vi "appendExptParam.vi"(8 "error in (no error)":errorcluster, 9 "value":variant, 10 "key":string, 11 "Inst.Transport in":refnum<class "Inst.Transport.lvclass">) -> (0 "error out":errorcluster, 3 "Inst.Transport out":refnum<class "Inst.Transport.lvclass">)   [LabVIEW 2019, in "Inst.Transport.lvclass"]
uses:
  Inst.Transport.lvclass
  Typedefs/Inst.Transport.PublicCommands--Enum.ctl
  e5f6a06c-75fd-45dd-8cd9-e6d3d0cfac2f.vi
  <vilib>/JDP Science/JSONtext/Variant to JSON Text.vi
  <vilib>/JDP Science/JSONtext/Set Item.vi
  <vilib>/JDP Science/JSONtext/LVClass Serializer/JSONtext LVClass Serializer.lvclass
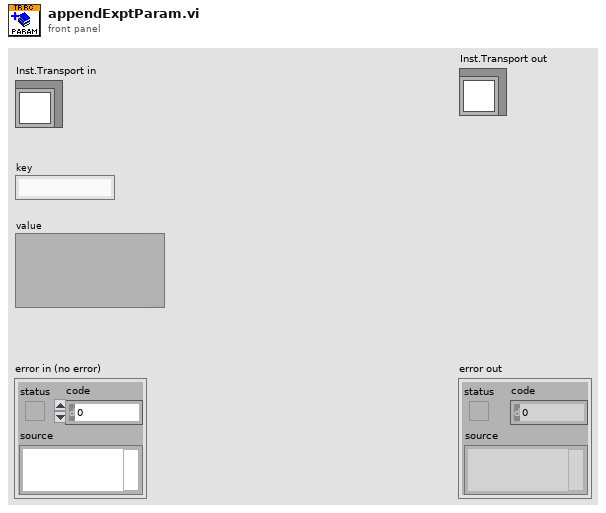
[diagram p1: front panel]
types:
  T1 = typedef "Inst.Transport.lvclass/Inst.Transport.PublicCommands--Enum.ctl" = enum16{"startTransport", "stopTransport", "getStatus", "setExptFolder", "setExptComments", "appendExptParam", "clearExptParam", "setExptParam", "setSweepConfig"}
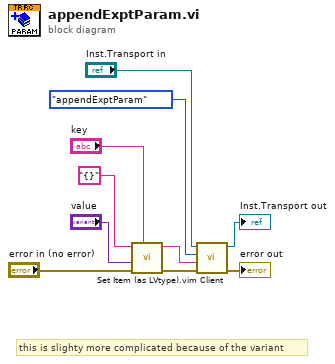
[diagram p0: block diagram]
diagram:
  # "this is slighty more complicated because of the variant"
  n1 = call "Set Item (as LVtype).vim"("$Path or Item Name"="key", "error in (no error)"="error in (no error)", "Anything"="value", "JSON"="{}") -> ("error out"=w1:errorcluster, "<JSON>"=w3:string)  [unwired: 4 in, 1 out]
  n2 = call-dynamic "Client.vi"("error in (no error)"=w1, "Data in"=w3, "Command in"=Inst.Transport.PublicCommands--Enum."appendExptParam" ("Commands"), "Instrument in"="Inst.Transport in") -> ("error out"=→"error out":errorcluster, "Instrument out"=→"Inst.Transport out":refnum<class "Inst.Transport.lvclass">)  [unwired: 4 in, 2 out]
